vi "Next.vi"(8 "error in (no error)":errorcluster, 11 "JSON Lexer in":refnum<class "JSON Lexer.lvclass">) -> (0 "error out":errorcluster, 1 "EOF":bool, 2 "Rune":string, 3 "JSON Lexer out":refnum<class "JSON Lexer.lvclass">)   [LabVIEW 2019, in "JKI JSON Serialization.lvlib" / "JSON Lexer.lvclass"]
doc: "JKI JSON 1.1.10.37\nTomi Maila - JKI\nCopyright (c) 2017, JKI"
uses:
  JSON Lexer.lvclass
  JSON Lexer.lvclass/JSON Lexer.ctl
  Unicode/UTF-8 String/UTF-8 String.lvclass/UTF-8 String.ctl
  Unicode/UTF-8 String/Next Rune As UTF-8 Substring.vi
  Unicode/UTF-8 String/Bytes In Rune.vi
  <vilib>/Utility/error.llb/Error Cluster From Error Code.vi
  Unicode/UTF-8 String/UTF-8 String.lvclass
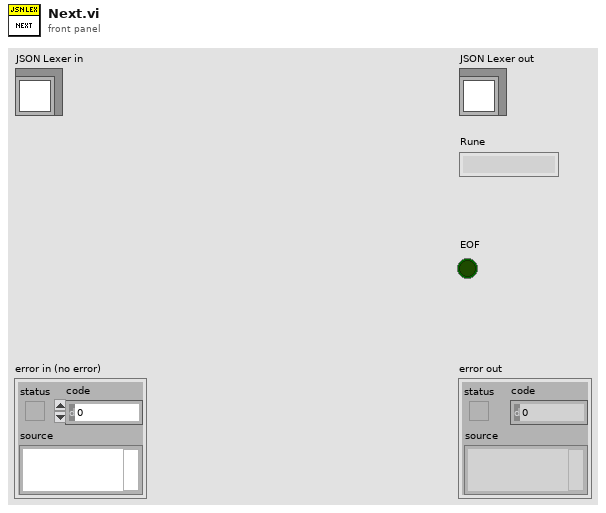
[diagram p1: front panel]
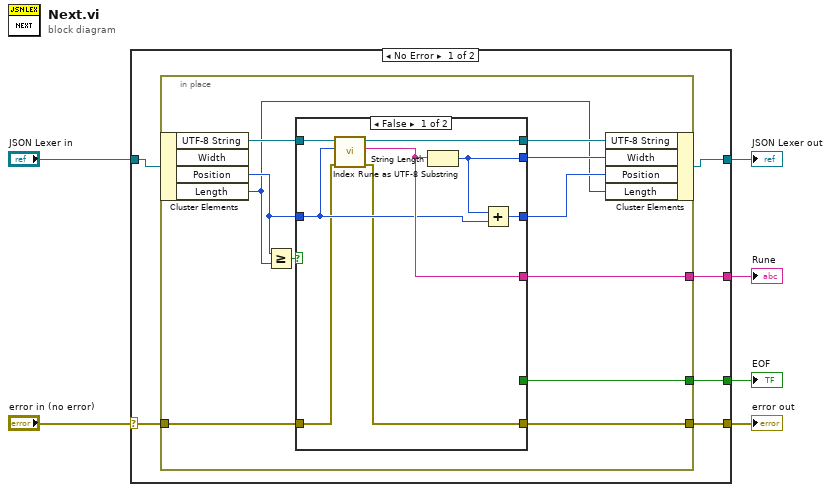
[diagram p0: block diagram]
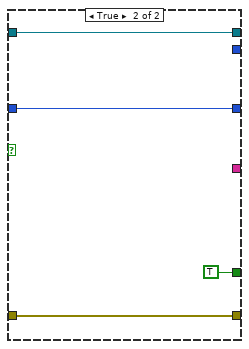
[diagram p2: hidden frame]
diagram:
  n1 = case shown="No Error" "error in (no error)" {
    selector: "error in (no error)" -> [w10 w37]
    tunnel: [w11 w37] -> w5
    tunnel: [w8 w36] -> w3
    tunnel: "JSON Lexer in" -> [w7 w36]
    tunnel: [w12 _] -> w2
    tunnel: [w9 _] -> w1
    frame No Error {
      n2 = in-place {
        in-place-border: [w16] -> w12
        in-place-border: [w23] -> w11
        in-place-border: w10 -> [w22]
        in-place-border: [w20] -> w9
        n3 = in-place-cluster #1(w7) -> ("UTF-8 String"=w18:refnum<class "UTF-8 String.lvclass">, "Position"=w15:i32, "Length"=w13:i32)  [unwired: 1 out]
        n4 = Greater Or Equal?(x=w15, y=w13) -> (x >= y?=w21:bool)
        n5 = case shown="False" w21 {
          tunnel: [w28 w35] -> w19
          tunnel: [w27 _] -> w14
          tunnel: [w29 _] -> w16
          tunnel: w15 -> [w26 w35]
          tunnel: [w24 w33] -> w23
          tunnel: w22 -> [w25 w33]
          tunnel: [_ TRUE] -> w20
          tunnel: w18 -> [w31 w32]
          tunnel: [w30 w32] -> w17
          frame False {
            n6 = call "Index Rune as UTF-8 Substring.vi"("error in (no error)"=w25, "Byte Offset"=w26, "UTF8 in"=w31) -> ("error out"=w24:errorcluster, "Rune"=w29:string, "UTF8 out"=w30:refnum<class "UTF-8 String.lvclass">)  [unwired: 6 in]
            n7 = String Length(string=w29) -> (length=w27:i32)
            n8 = Add(x=w27, y=w26) -> (x+y=w28:i32)
          }
          frame True {
          }
        }
        n9 = in-place-cluster #1("UTF-8 String"=w17, "Width"=w14, "Position"=w19, "Length"=w13) -> (w8:refnum<class "JSON Lexer.lvclass">)
      }
    }
    frame Error {
    }
  }
  "error out" <- w5
  "JSON Lexer out" <- w3
  "Rune" <- w2
  "EOF" <- w1
